vi "SSH Async Execute Command.vi"(8 "Error In":errorcluster, 10 "Command":string, 11 "Install LV Data in":T1) -> (0 "Error Out":errorcluster, 3 "Install LV Data out":T1)   [LabVIEW 2011, in "LMH-LINX.lvlib"]
uses:
  LMH-LINX.lvlib
  Target Management/Install LV Data.ctl
  C:/Users/samkristoff/Desktop/Builds/2016_01_27/build/LabVIEW/vi.lib/MakerHub/LINX/Resources/Renci.SshNet.dll
  Resources/Renci.SshNet.dll
  Target Management/Target Info.ctl
  Target Management/NIC Info.ctl
  Target Management/NIC Mode.ctl
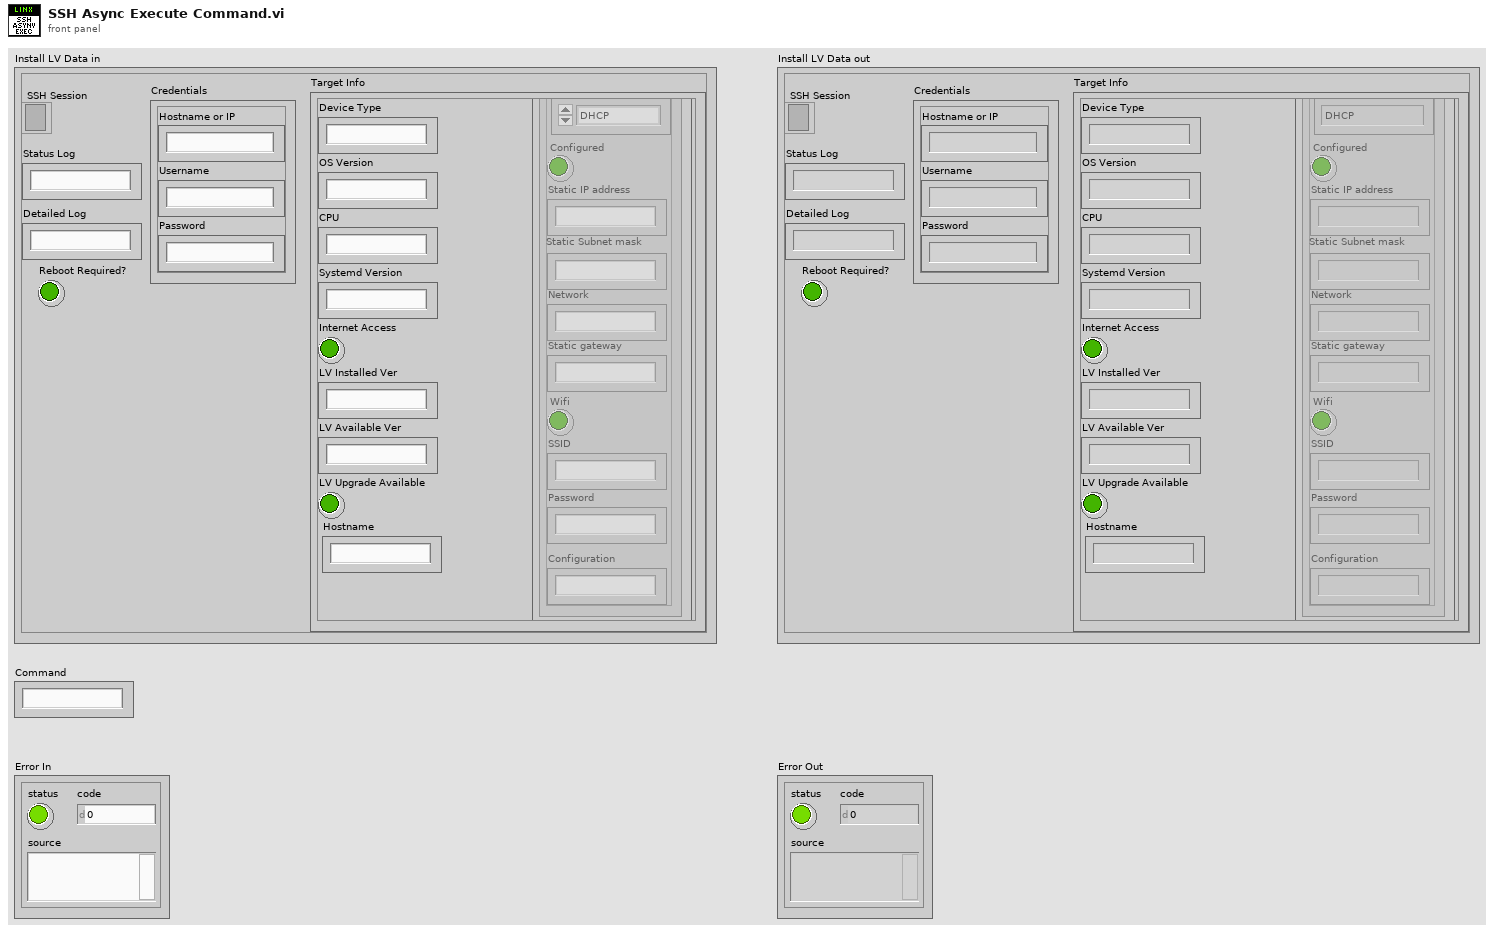
[diagram p1: front panel]
types:
  T1 = typedef "LMH-LINX.lvlib/Install LV Data.ctl" = cluster{"SSH Session":refnum<k24>, "Status Log":string, "Detailed Log":string, "Credentials":cluster{"Hostname or IP":string, "Username":string, "Password":string}, "Target Info":T2, "Reboot Required?":bool}
  T2 = typedef "LMH-LINX.lvlib/Target Info.ctl" = cluster{"OS Version":string, "CPU":string, "Systemd Version":string, "Internet Access":bool, "Device Type":string, "LV Installed Ver":string, "LV Available Ver":string, "LV Upgrade Available":bool, "Hostname":string, "NIC Info":T3[]}
  T3 = typedef "LMH-LINX.lvlib/NIC Info.ctl" = cluster{"Name":string, "NIC Mode":T4, "Configured":bool, "Static IP address":string, "Static Subnet mask":string, "Network":string, "Static gateway":string, "Wifi":bool, "SSID":string, "Password":string, "Configuration":string}
  T4 = typedef "LMH-LINX.lvlib/NIC Mode.ctl" = enum16{"DHCP", "Static", "Loopback"}
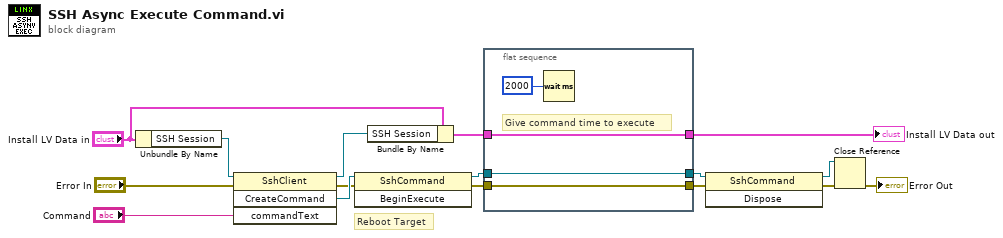
[diagram p0: block diagram]
diagram:
  # "Reboot Target"
  n1 = Unbundle By Name("Install LV Data in") -> ("SSH Session"=w4:refnum<k24>)
  n2 = invoke class="SshClient" method="CreateCommand"(reference=w4, error in="Error In", "commandText"="Command") -> (reference out=w5:refnum<k24>, error out=w8:errorcluster, "CreateCommand"=w11:refnum<k24>)  [unwired: 1 in, 1 out]
  n3 = invoke class="SshCommand" method="BeginExecute"(reference=w11, error in=w8) -> (reference out=w13:refnum<k24>, error out=w10:errorcluster)  [unwired: 1 in, 1 out]
  n4 = Bundle By Name(cluster="Install LV Data in", "SSH Session"=w5) -> (w15:T1)
  n5 = flat-sequence {
    tunnel: [w19] -> w9
    tunnel: w10 -> [w19]
    tunnel: [w18] -> w12
    tunnel: w13 -> [w18]
    tunnel: [w17] -> w14
    tunnel: w15 -> [w17]
    frame #0 {
      # "Give command time to execute"
      n6 = Wait (ms)(milliseconds to wait=u32 2000) -> ()  [unwired: 1 out]
    }
  }
  n7 = invoke class="SshCommand" method="Dispose"(reference=w12, error in=w9) -> (reference out=w3:refnum<k24>, error out=w2:errorcluster)  [unwired: 1 in, 1 out]
  n8 = Close Reference(reference=w3, error in (no error)=w2) -> (error out=→"Error Out":errorcluster)
  "Install LV Data out" <- w14
